vi "PFinal.vi"() -> ()   [LabVIEW 2020]
uses:
  <vilib>/Instr/_visa.llb/VISA Configure Serial Port (Instr).vi
  <vilib>/httpClient/PUTBuffer.vi
  <vilib>/httpClient/LabVIEWHTTPClient.lvlib
panel:
  in  "VISA resource name":refnum<visa-resource-name>
  in  "Stop":bool
  in  "Tab Control":enum32{"Manual", "Jade", "Snake"}(tab)
  out "Dist":dbl
  out "Hum":dbl
  out "Nivel de agua":dbl(slide) scale=0.0..30.0
  out "Humedad":dbl(knob) scale=0.0..100.0
  out "Temp":dbl
  out "Temperatura":dbl(slide) scale=0.0..100.0
  in  "Color":bool
  in  "Encender Led":bool
  in  "Bomba":bool
  in  "Ventilador":bool
  out "Dist":dbl
  out "Hum":dbl
  out "Nivel de agua":dbl(slide) scale=0.0..30.0
  out "Humedad":dbl(knob) scale=0.0..100.0
  out "Temp":dbl
  out "Temperatura":dbl(slide) scale=0.0..100.0
  in  "Color":bool
  in  "Encender Led":bool
  out "Bomba":bool
  out "Alarma de agua":bool
  out "Ventilador":bool
  out "Dist":dbl
  out "Hum":dbl
  out "Nivel de agua":dbl(slide) scale=0.0..30.0
  out "Humedad":dbl(knob) scale=0.0..100.0
  out "Temp":dbl
  out "Temperatura":dbl(slide) scale=0.0..100.0
  in  "Color":bool
  out "Bomba":bool
  out "Alarma":bool
  in  "Encender Led":bool
  out "Ventilador":bool
  in  "Modo":u16(ring) items=["Manual", "Jade", "Snake"]
  # "Sistema de Mantenimiento de plantas"
  # "Rojo"
  # "Azul"
  # "Rojo"
  # "Azul"
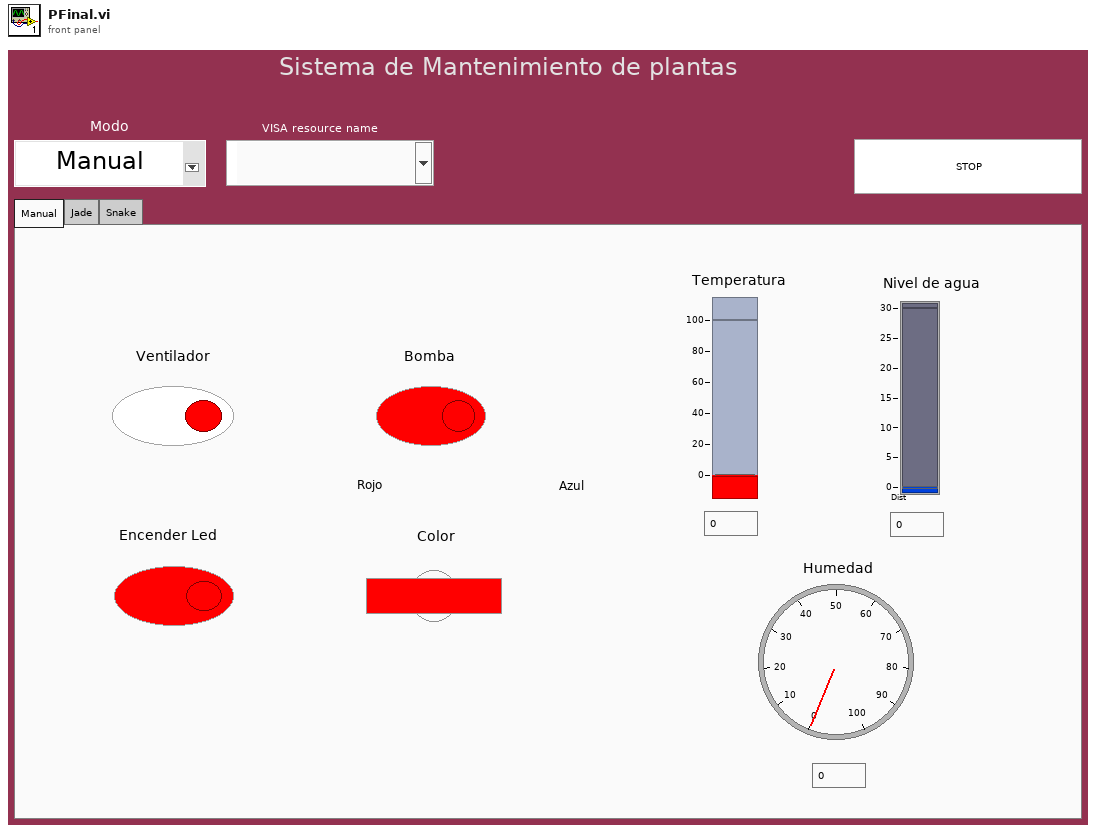
[diagram p1: front panel]
types:
  T1 = cluster{"Planta":string, "Data":string, "Hora":string, "Temperatura":dbl, "Humedad":dbl, "Distancia":dbl}
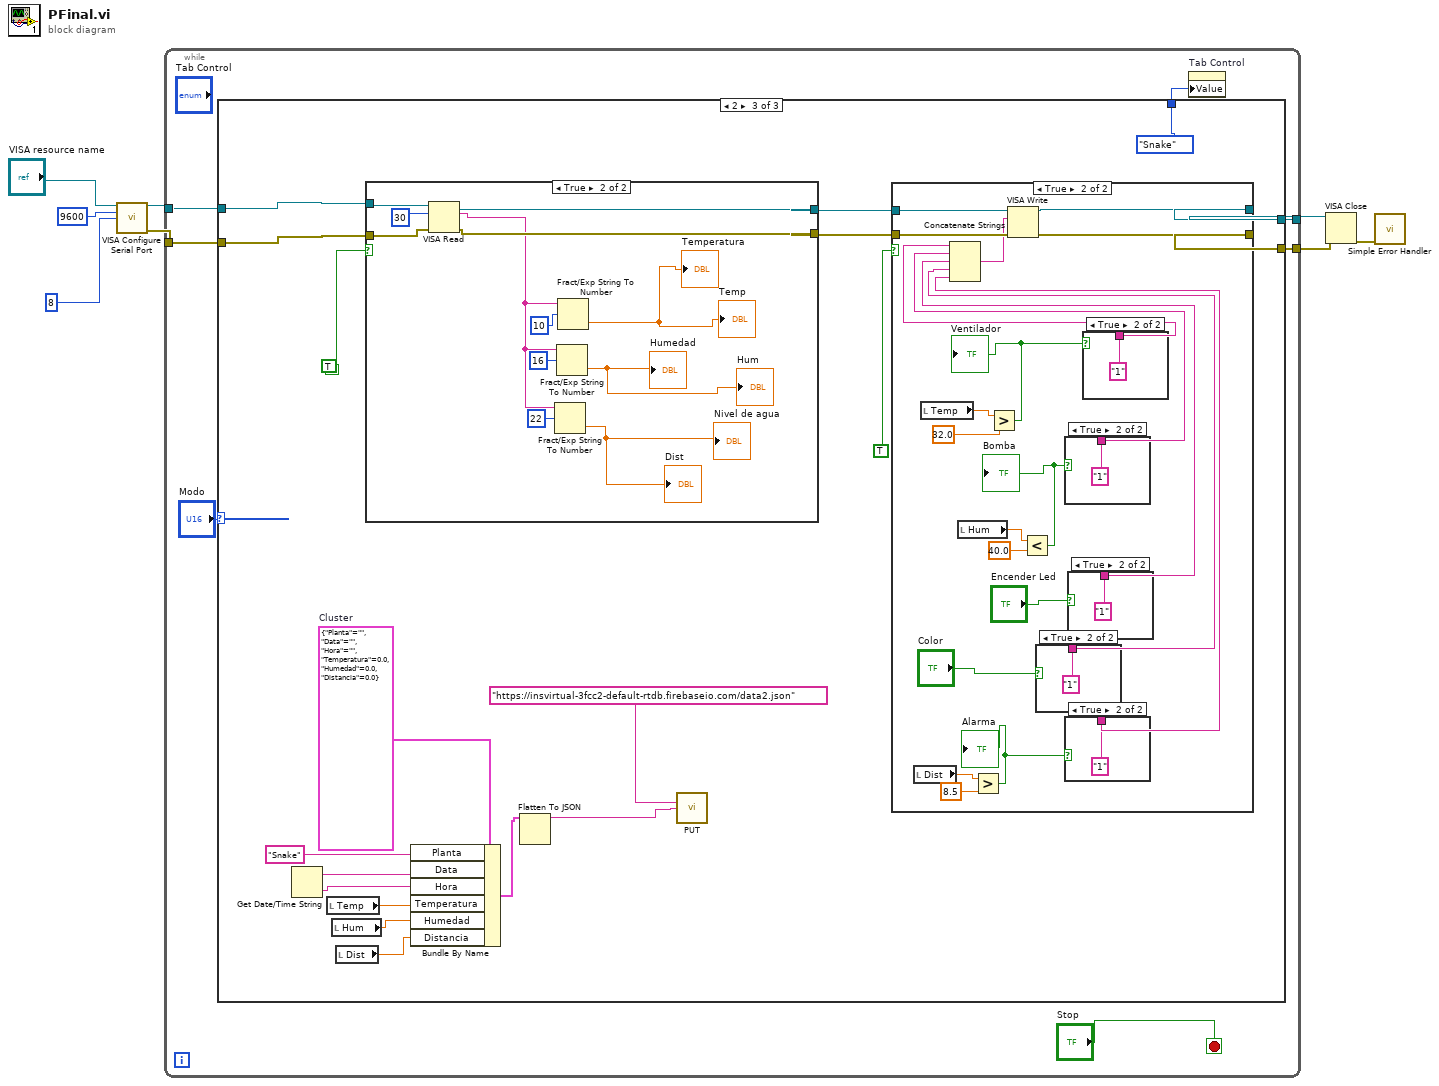
[diagram p0: block diagram]
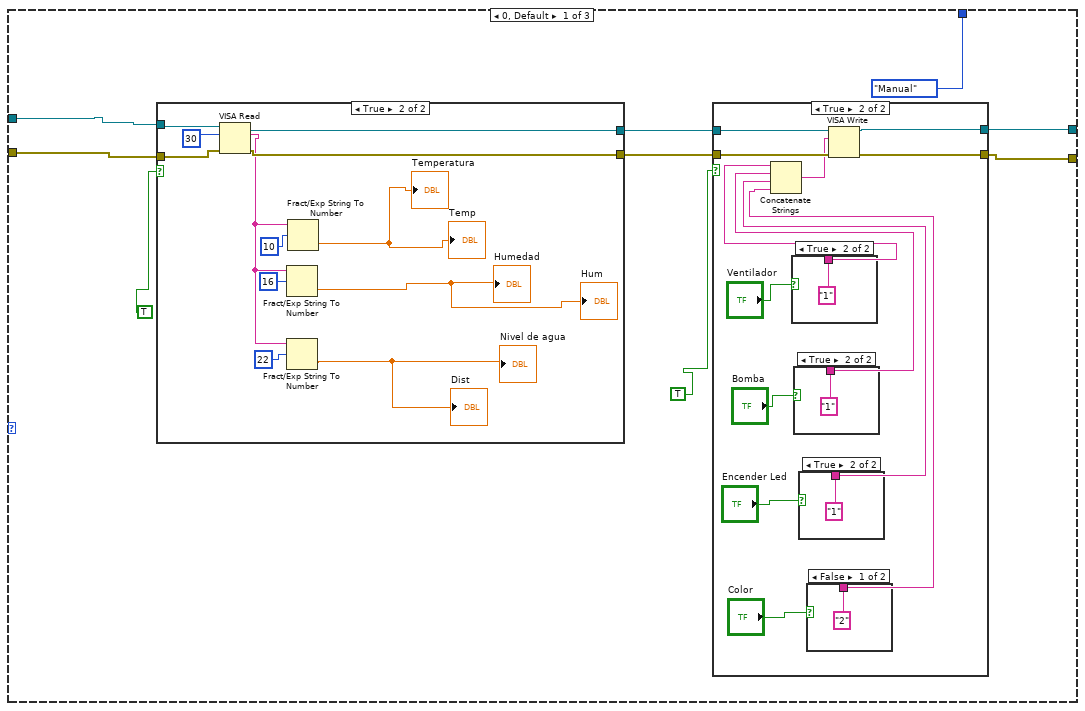
[diagram p2: hidden frame]
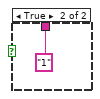
[diagram p4: hidden frame]
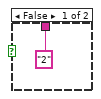
[diagram p5: hidden frame]
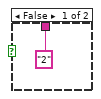
[diagram p6: hidden frame]
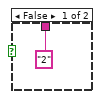
[diagram p7: hidden frame]
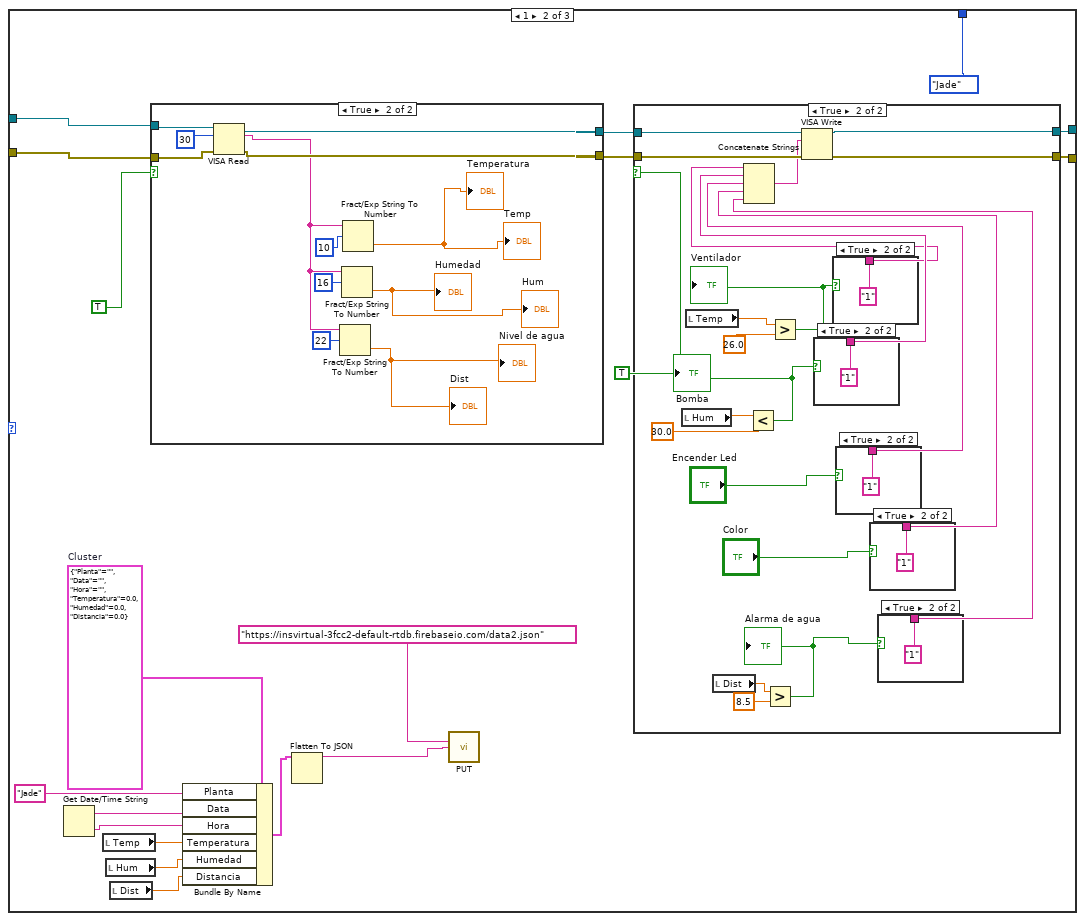
[diagram p9: hidden frame]
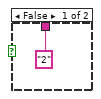
[diagram p11: hidden frame]
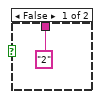
[diagram p12: hidden frame]
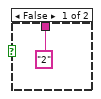
[diagram p13: hidden frame]
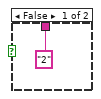
[diagram p14: hidden frame]
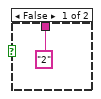
[diagram p15: hidden frame]
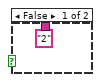
[diagram p18: hidden frame]
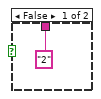
[diagram p19: hidden frame]
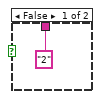
[diagram p20: hidden frame]
diagram:
  n1 = call-poly "VISA Configure Serial Port"("VISA resource name"="VISA resource name", "baud rate (9600)"=u32 9600, "data bits (8)"=u16 8) -> ("VISA resource name out"=w6:refnum<visa-resource-name>, "error out"=w5:errorcluster)  [unwired: 11 in]
  n2 = while {
    tunnel: w6 -> [w15]
    tunnel: w5 -> [w14]
    tunnel: [w13] -> w3
    tunnel: [w12] -> w2
    stop <- "Stop" stop-if-true
    n3 = case shown="2" "Modo" {
      tunnel: w15 -> [w22 w77 w142]
      tunnel: w14 -> [w21 w76 w143]
      tunnel: [w20 w75 w141] -> w13
      tunnel: [w19 w74 w140] -> w12
      tunnel: [enum32{"Manual", "Jade", "Snake"}."Manual" ("Tab Control") enum32{"Manual", "Jade", "Snake"}."Jade" ("Tab Control") enum32{"Manual", "Jade", "Snake"}."Snake" ("Tab Control")] -> w9
      frame 0, Default {
        n4 = case shown="True" TRUE {
          tunnel: w22 -> [w49 w61]
          tunnel: w21 -> [w48 w60]
          tunnel: [w49 w58] -> w23
          tunnel: [w48 w57] -> w24
          frame False {
          }
          frame True {
            n5 = VISA Read(VISA resource name=w61, byte count=u32 30, error in (no error)=w60) -> (VISA resource name out=w58:refnum<visa-resource-name>, read buffer=w52:string, error out=w57:errorcluster)  [unwired: 1 out]
            n6 = Fract/Exp String To Number(string=w52, offset=16) -> (number=→"Humedad" →"Hum":dbl)  [unwired: 2 in, 1 out]
            n7 = Fract/Exp String To Number(string=w52, offset=22) -> (number=→"Nivel de agua" →"Dist":dbl)  [unwired: 2 in, 1 out]
            n8 = Fract/Exp String To Number(string=w52, offset=10) -> (number=→"Temperatura" →"Temp":dbl)  [unwired: 2 in, 1 out]
          }
        }
        n9 = case shown="True" TRUE {
          tunnel: w23 -> [w26 w39]
          tunnel: w24 -> [w25 w38]
          tunnel: [w26 w37] -> w20
          tunnel: [w25 w36] -> w19
          frame False {
          }
          frame True {
            n10 = case shown="True" "Ventilador" {
              tunnel: ["2" ("write buffer") "1" ("write buffer")] -> w34
              frame False {
              }
              frame True {
              }
            }
            n11 = case shown="True" "Bomba" {
              tunnel: ["2" ("write buffer") "1" ("write buffer")] -> w35
              frame False {
              }
              frame True {
              }
            }
            n12 = case shown="True" "Encender Led" {
              tunnel: ["2" ("write buffer") "1" ("write buffer")] -> w32
              frame False {
              }
              frame True {
              }
            }
            n13 = case shown="False" "Color" {
              tunnel: ["2" ("write buffer") "1" ("write buffer")] -> w31
              frame False {
              }
              frame True {
              }
            }
            n14 = Concatenate Strings(w34, w35, w32, w31) -> (w33:string)
            n15 = VISA Write(VISA resource name=w39, write buffer=w33, error in (no error)=w38) -> (VISA resource name out=w37:refnum<visa-resource-name>, error out=w36:errorcluster)  [unwired: 1 out]
          }
        }
      }
      frame 1 {
        w63 = T1 {"Planta"="", "Data"="", "Hora"="", "Temperatura"=0.0, "Humedad"=0.0, "Distancia"=0.0}  # Cluster
        n16 = Get Date/Time String() -> (date string=w68:string, time string=w67:string)  [unwired: 3 in]
        n17 = local read "Temp"() -> (w64:dbl)
        n18 = local read "Hum"() -> (w65:dbl)
        n19 = local read "Dist"() -> (w66:dbl)
        n20 = case shown="True" TRUE {
          tunnel: w77 -> [w115 w127]
          tunnel: w76 -> [w114 w126]
          tunnel: [w115 w124] -> w78
          tunnel: [w114 w123] -> w79
          frame False {
          }
          frame True {
            n21 = VISA Read(VISA resource name=w127, byte count=u32 30, error in (no error)=w126) -> (VISA resource name out=w124:refnum<visa-resource-name>, read buffer=w118:string, error out=w123:errorcluster)  [unwired: 1 out]
            n22 = Fract/Exp String To Number(string=w118, offset=22) -> (number=→"Nivel de agua" →"Dist":dbl)  [unwired: 2 in, 1 out]
            n23 = Fract/Exp String To Number(string=w118, offset=16) -> (number=→"Humedad" →"Hum":dbl)  [unwired: 2 in, 1 out]
            n24 = Fract/Exp String To Number(string=w118, offset=10) -> (number=→"Temperatura" →"Temp":dbl)  [unwired: 2 in, 1 out]
          }
        }
        n25 = Bundle By Name(cluster=w63, "Planta"="Jade", "Data"=w68, "Hora"=w67, "Temperatura"=w64, "Humedad"=w65, "Distancia"=w66) -> (w62:T1)
        n26 = Flatten To JSON(anything=w62) -> (JSON string=w71:string)  [unwired: 2 in, 1 out]
        n27 = call-poly <vilib>:"PUT.vi"("url"="https://insvirtual-3fcc2-default-rtdb.firebaseio.com/data2.json", "buffer"=w71) -> ()  [unwired: 10 in, 4 out]
        n28 = case shown="True" TRUE {
          tunnel: w78 -> [w82 w103]
          tunnel: w79 -> [w81 w102]
          tunnel: [w82 w101] -> w75
          tunnel: [w81 w100] -> w74
          frame False {
          }
          frame True {
            n29 = local read "Hum"() -> (w88:dbl)
            n30 = local read "Temp"() -> (w91:dbl)
            n31 = local read "Dist"() -> (w85:dbl)
            n32 = Less?(x=w88, y=30.0) -> (x < y?=w86:bool)
            "Bomba" <- w86
            n33 = Greater?(x=w85, y=8.5) -> (0:w83:bool)
            "Alarma de agua" <- w83
            n34 = Greater?(x=w91, y=26.0) -> (0:w89:bool)
            "Ventilador" <- w89
            n35 = case shown="True" w86 {
              tunnel: ["2" ("write buffer") "1" ("write buffer")] -> w99
              frame False {
              }
              frame True {
              }
            }
            n36 = case shown="True" w89 {
              tunnel: ["2" ("write buffer") "1" ("write buffer")] -> w98
              frame False {
              }
              frame True {
              }
            }
            n37 = case shown="True" "Encender Led" {
              tunnel: ["2" ("write buffer") "1" ("write buffer")] -> w96
              frame False {
              }
              frame True {
              }
            }
            n38 = case shown="True" "Color" {
              tunnel: ["2" ("write buffer") "1" ("write buffer")] -> w95
              frame False {
              }
              frame True {
              }
            }
            n39 = case shown="True" w83 {
              tunnel: ["2" ("write buffer") "1" ("write buffer")] -> w94
              frame False {
              }
              frame True {
              }
            }
            n40 = Concatenate Strings(w98, w99, w96, w95, w94) -> (w97:string)
            n41 = VISA Write(VISA resource name=w103, write buffer=w97, error in (no error)=w102) -> (VISA resource name out=w101:refnum<visa-resource-name>, error out=w100:errorcluster)  [unwired: 1 out]
          }
        }
      }
      frame 2 {
        w129 = T1 {"Planta"="", "Data"="", "Hora"="", "Temperatura"=0.0, "Humedad"=0.0, "Distancia"=0.0}  # Cluster
        n42 = Get Date/Time String() -> (date string=w134:string, time string=w133:string)  [unwired: 3 in]
        n43 = local read "Temp"() -> (w132:dbl)
        n44 = local read "Hum"() -> (w131:dbl)
        n45 = local read "Dist"() -> (w130:dbl)
        n46 = case shown="True" TRUE {
          tunnel: w142 -> [w181 w193]
          tunnel: w143 -> [w180 w192]
          tunnel: [w181 w190] -> w144
          tunnel: [w180 w189] -> w145
          frame False {
          }
          frame True {
            n47 = VISA Read(VISA resource name=w193, byte count=u32 30, error in (no error)=w192) -> (VISA resource name out=w190:refnum<visa-resource-name>, read buffer=w184:string, error out=w189:errorcluster)  [unwired: 1 out]
            n48 = Fract/Exp String To Number(string=w184, offset=22) -> (number=→"Nivel de agua" →"Dist":dbl)  [unwired: 2 in, 1 out]
            n49 = Fract/Exp String To Number(string=w184, offset=16) -> (number=→"Humedad" →"Hum":dbl)  [unwired: 2 in, 1 out]
            n50 = Fract/Exp String To Number(string=w184, offset=10) -> (number=→"Temperatura" →"Temp":dbl)  [unwired: 2 in, 1 out]
          }
        }
        n51 = Bundle By Name(cluster=w129, "Planta"="Snake", "Data"=w134, "Hora"=w133, "Temperatura"=w132, "Humedad"=w131, "Distancia"=w130) -> (w128:T1)
        n52 = Flatten To JSON(anything=w128) -> (JSON string=w137:string)  [unwired: 2 in, 1 out]
        n53 = call-poly <vilib>:"PUT.vi"("url"="https://insvirtual-3fcc2-default-rtdb.firebaseio.com/data2.json", "buffer"=w137) -> ()  [unwired: 10 in, 4 out]
        n54 = case shown="True" TRUE {
          tunnel: w144 -> [w148 w169]
          tunnel: w145 -> [w147 w168]
          tunnel: [w148 w167] -> w141
          tunnel: [w147 w166] -> w140
          frame False {
          }
          frame True {
            n55 = local read "Dist"() -> (w151:dbl)
            n56 = local read "Temp"() -> (w157:dbl)
            n57 = local read "Hum"() -> (w153:dbl)
            n58 = Greater?(x=w151, y=8.5) -> (0:w149:bool)
            "Alarma" <- w149
            n59 = Greater?(x=w157, y=32.0) -> (0:w155:bool)
            "Ventilador" <- w155
            n60 = Less?(x=w153, y=40.0) -> (x < y?=w152:bool)
            "Bomba" <- w152
            n61 = case shown="True" "Color" {
              tunnel: ["2" ("write buffer") "1" ("write buffer")] -> w161
              frame False {
              }
              frame True {
              }
            }
            n62 = case shown="True" w152 {
              tunnel: ["2" ("write buffer") "1" ("write buffer")] -> w165
              frame False {
              }
              frame True {
              }
            }
            n63 = case shown="True" w149 {
              tunnel: ["2" ("write buffer") "1" ("write buffer")] -> w160
              frame False {
              }
              frame True {
              }
            }
            n64 = case shown="True" "Encender Led" {
              tunnel: ["2" ("write buffer") "1" ("write buffer")] -> w162
              frame False {
              }
              frame True {
              }
            }
            n65 = case shown="True" w155 {
              tunnel: ["2" ("write buffer") "1" ("write buffer")] -> w164
              frame False {
              }
              frame True {
              }
            }
            n66 = Concatenate Strings(w164, w165, w162, w161, w160) -> (w163:string)
            n67 = VISA Write(VISA resource name=w169, write buffer=w163, error in (no error)=w168) -> (VISA resource name out=w167:refnum<visa-resource-name>, error out=w166:errorcluster)  [unwired: 1 out]
          }
        }
      }
    }
    n68 = property on="Tab Control" class="TabCtl (strict)"("Value"=w9) -> ()  [unwired: 2 in, 2 out]
  }
  n69 = VISA Close(VISA resource name=w3, error in (no error)=w2) -> (error out=w4:errorcluster)
  n70 = call <vilib>:"Simple Error Handler.vi"("error in (no error)"=w4) -> ()  [unwired: 4 in, 5 out]
